vi "Untitled 8.vi"() -> ()   [LabVIEW 2023]
panel:
  out "shortcut":bool
  out "directory":bool
  out "resolved path":path
  out "path out":path
  out "size":i64
  out "last mod":timestamp
  out "error out":errorcluster
  in  "path":path
  in  "error in":errorcluster
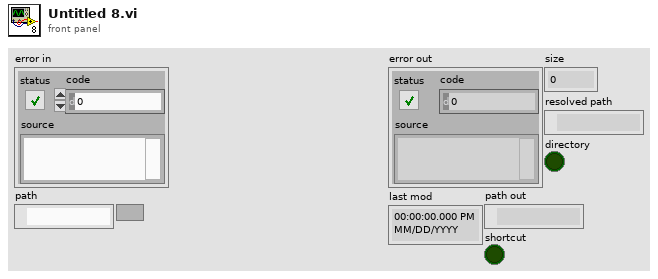
[diagram p1: front panel]
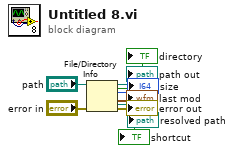
[diagram p0: block diagram]
diagram:
  n1 = File/Directory Info(path="path", error in="error in") -> (path out=→"path out":path, directory=→"directory":bool, size=→"size":i64, last mod=→"last mod":timestamp, error out=→"error out":errorcluster, resolved path=→"resolved path":path, shortcut=→"shortcut":bool)
